vi "Get Name.vi"(8 "error in (no error)":errorcluster {"code" format="Error %.0f"}, 11 "Library Documentation In":refnum<class "Library Documentation.lvclass">) -> (0 "error out":errorcluster {"code" format="Error %.0f"}, 2 "Name":string, 3 "Library Documentation Out":refnum<class "Library Documentation.lvclass">)   [LabVIEW 2023, in "VIDoc Parsing.lvlib" / "Library Documentation.lvclass"]
uses:
  Library Documentation.lvclass
  Library Documentation.lvclass/Library Documentation.ctl
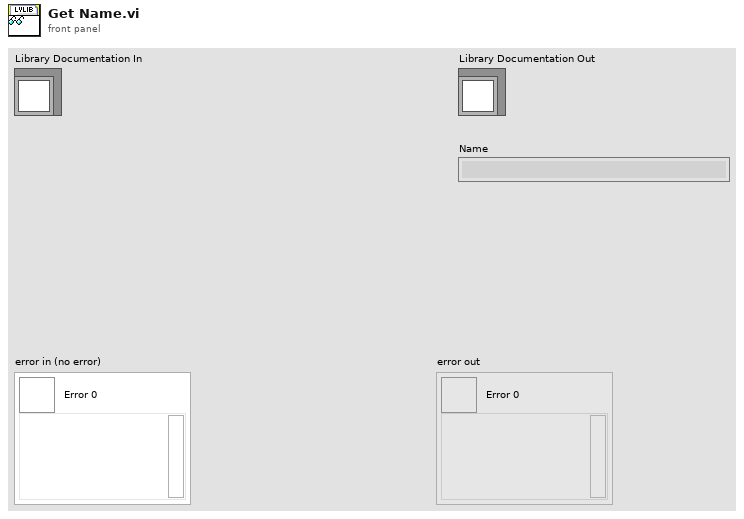
[diagram p1: front panel]
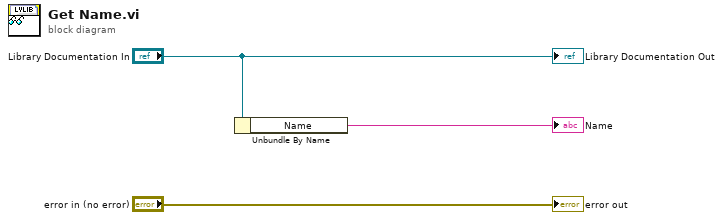
[diagram p0: block diagram]
diagram:
  n1 = Unbundle By Name("Library Documentation In") -> ("Name"=→"Name":string)
  "error out" <- "error in (no error)"
  "Library Documentation Out" <- "Library Documentation In"
